vi "FetchCalibration.vi"(8 "error in (no error)":errorcluster, 10 "instruments":string[](array[string]), 11 "ByteQXAPIBase in":refnum<class "ByteQXAPIBase.lvclass">) -> (0 "error out":errorcluster, 2 "instruments":T1[](array[typedef]), 3 "ByteQXAPIBase out":refnum<class "ByteQXAPIBase.lvclass">)   [LabVIEW 2019, in "ByteQXWebAPI.lvlib" / "ByteQXAPIBase.lvclass"]
doc: "Obtain instruments calibrations based on the Instrument Slug"
uses:
  ByteQXAPIBase.lvclass
  Converted_Slug_Cluster.ctl
  <vilib>/Bytelabs/ByteREST/ByteRESTClass/ByteRESTBase/HTTP/Status_Code.ctl
  JSON_Slug_Cluster.ctl
  Private/module.ctl
  ByteQXAPIBase.lvclass/ByteQXAPIBase.ctl
  <vilib>/Bytelabs/ByteREST/ByteRESTClass/ByteRESTBase/RESTBase.lvclass
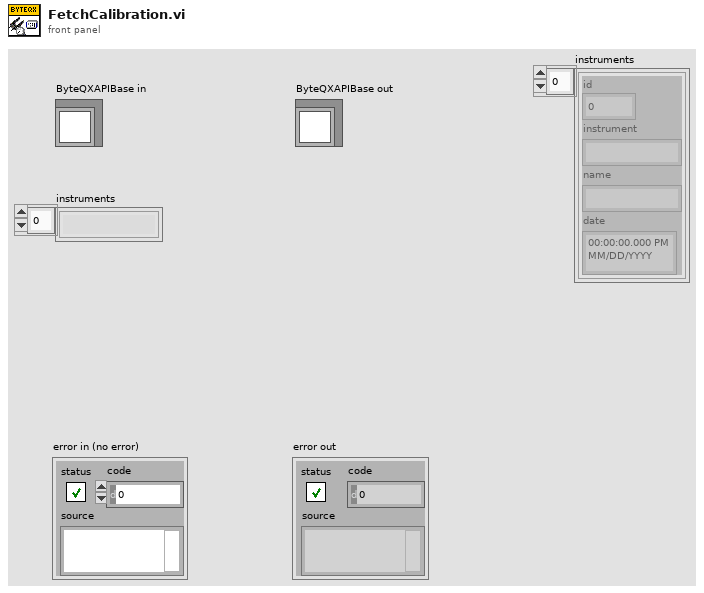
[diagram p1: front panel]
types:
  T1 = typedef "ByteQXWebAPI.lvlib/ByteQXAPIBase.lvclass/Converted_Slug_Cluster.ctl" = cluster{"id":u32, "instrument":string, "name":string, "date":timestamp}
  T2 = typedef "ByteQXWebAPI.lvlib/ByteQXAPIBase.lvclass/module.ctl" = enum16{"gs", "tms"}
  T3 = typedef "ByteQXWebAPI.lvlib/ByteQXAPIBase.lvclass/JSON_Slug_Cluster.ctl" = cluster{"id":u32, "instrument":string, "name":string, "data":string}
  T4 = typedef "ByteREST.lvlib/RESTBase.lvclass/Status_Code.ctl" = u16
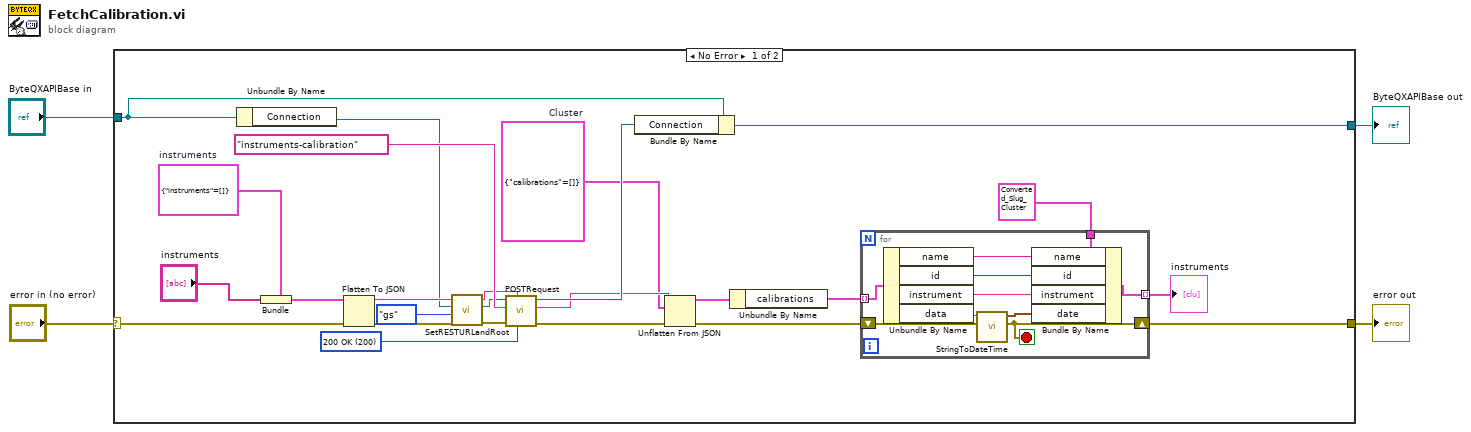
[diagram p0: block diagram]
diagram:
  n1 = case shown="No Error" "error in (no error)" {
    selector: "error in (no error)" -> [w24 w40]
    tunnel: [w17 w40] -> w3
    tunnel: [w27 w39] -> w1
    tunnel: "ByteQXAPIBase in" -> [w28 w39]
    frame No Error {
      w11 = cluster{"calibrations":T3[]} {"calibrations"=[]}  # Cluster
      w16 = cluster{"instruments":string[]} {"instruments"=[]}  # instruments
      w21 = T4 200 items=["200 OK"=200, "201 Created"=201, "400 Bad Request"=400, "401 Unauthorized"=401, "403 Forbidden"=403, "404 Not Found"=404, "405 Method Not Allowed"=405, "406 Not Acceptable"=406, "500 Internal Server Error"=500] ("expected response")
      n2 = Unbundle By Name(w28) -> ("Connection"=w7:refnum<class "RESTBase.lvclass">)
      n3 = Bundle(cluster=w16, "instruments"="instruments") -> (w14:cluster{"instruments":string[]})
      n4 = Flatten To JSON(anything=w14, error in (no error)=w24) -> (JSON string=w20:string, 11:w9:errorcluster)  [unwired: 1 in]
      n5 = call "SetRESTURLandRoot.vi"("error in (no error)"=w9, "module"=module."gs", "ByteREST in"=w7) -> ("error out"=w8:errorcluster, "ByteREST out"=w6:refnum<class "RESTBase.lvclass">)  [unwired: 7 in]
      n6 = call-dynamic "POSTRequest.vi"("expected response"=w21, "Body in"=w20, "error in (no error)"=w8, "Request"="instruments-calibration", "ByteRESTBase in"=w6) -> ("error out"=w22:errorcluster, "Body"=w23:string, "ByteRESTBase out"=w26:refnum<class "RESTBase.lvclass">)  [unwired: 3 in, 1 out]
      n7 = Bundle By Name(cluster=w28, "Connection"=w26) -> (w27:refnum<class "ByteQXAPIBase.lvclass">)
      n8 = Unflatten From JSON(JSON string=w23, type and defaults=w11, error in (no error)=w22) -> (value=w19:cluster{"calibrations":T3[]}, error out=w18:errorcluster)  [unwired: 4 in]
      n9 = Unbundle By Name(w19) -> ("calibrations"=w13:T3[])
      n10 = for {
        tunnel: w13 -> [w38] mode=indexing
        tunnel: [w33] -> w12 mode=indexing
        tunnel: T1 {"id"=0, "instrument"="", "name"="", "date"=timestamp(0 s since 1904-01-01)} ("Converted_Slug_Cluster") -> [w30]
        shift-right: [w31] -> w17
        shift-left: w18 -> [w32]
        stop <- w31 stop-if-true
        n11 = Unbundle By Name(w38) -> ("name"=w29:string, "id"=w37:u32, "instrument"=w34:string, "data"=w36:string)
        n12 = call "StringToDateTime.vi"("error in (no error)"=w32, "datetime string"=w36) -> ("error out"=w31:errorcluster, "timestamp"=w35:timestamp)  [unwired: 8 in]
        n13 = Bundle By Name(cluster=w30, "name"=w29, "id"=w37, "instrument"=w34, "date"=w35) -> (w33:T1)
      }
      "instruments" <- w12
    }
    frame Error {
    }
  }
  "error out" <- w3
  "ByteQXAPIBase out" <- w1
